vi "3458A Select Aperture.vi"(1 "manual aperture [s]":dbl=1.4e-06 format="%#_6p", 2 "sampling rate [Sa/s]":dbl=10000.0, 3 "digitizer session":T1 {"channels"."Range [Vpk]" min=0.0}) -> (0 "selected aperture [s]":dbl format="%#_6p")   [LabVIEW 2018, in "3458A Virtual Digitizer.lvlib"]
doc: "Auto selection of aperture (if enabled in session!). Otherwise returns input aperture."
uses:
  3458A Virtual Digitizer.lvlib
  3458A Digitizer Session.ctl
  3458A Virtual Channel Config.ctl
  Counter/Counter Session.ctl
  Counter/Counter Type.ctl
  AWG/AWG Session.ctl
  AWG/AWG Type.ctl
  3458A Sync Mode.ctl
  3458A Idn Mode.ctl
  3458A Digitizing Low Levels/Configure/Sampling Mode.ctl
  3458A Digitizing Process Options.ctl
  3458A Data Packet.ctl
  3458A Aux Record Data.ctl
  3458A Digitizing Low Levels/Configure/Level Setup.ctl
  3458A Digitizing Low Levels/Configure/First Sample Trigger.ctl
  3458A Aperture Selection Mode.ctl
  3458A Digitizing Low Levels/3458A Digitizing Low Levels.lvlib
  Counter/Counter.lvlib
  AWG/AWG.lvlib
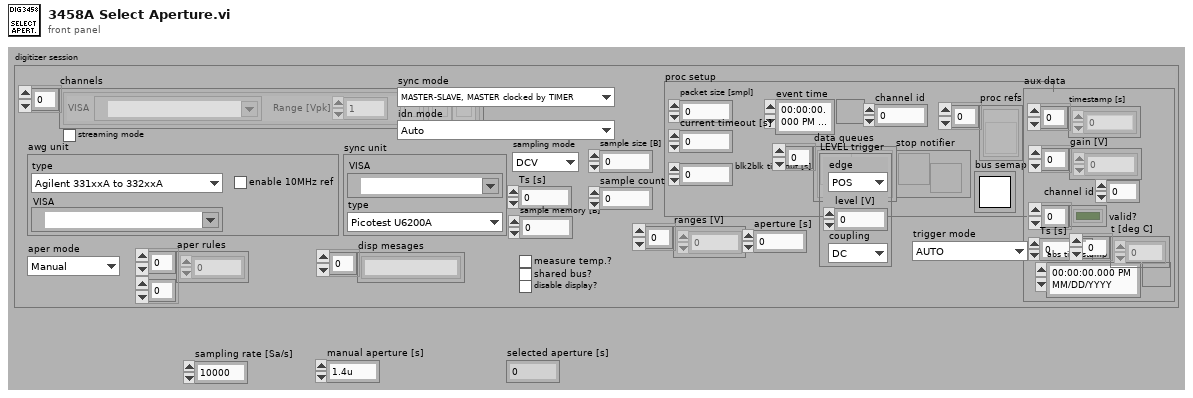
[diagram p1: front panel]
types:
  T1 = typedef "3458A Virtual Digitizer.lvlib/3458A Digitizer Session.ctl" = cluster{"channels":T2[], "sync unit":T3, "awg unit":T5, "sync mode":T7, "streaming mode":bool, "idn mode":T8, "sampling mode":T9, "Ts [s]":dbl, "sample memory [B]":i32, "proc setup":T10, "sample size [B]":i32, "sample count":i32, "aux data":T12, "ranges [V]":dbl[], "aperture [s]":dbl, "LEVEL trigger":T13, "trigger mode":T14, "measure temp.?":bool, "disp mesages":string[], "shared bus?":bool, "disable display?":bool, "aper mode":T15, "aper rules":dbl[][]}
  T2 = typedef "3458A Virtual Digitizer.lvlib/3458A Virtual Channel Config.ctl" = cluster{"VISA":refnum<visa-resource-name>, "Range [Vpk]":dbl, "btn clr":bool, "btn up":bool, "btn down":bool}
  T3 = typedef "Counter.lvlib/Counter Session.ctl" = cluster{"VISA":refnum<visa-resource-name>, "type":T4}
  T4 = typedef "Counter.lvlib/Counter Type.ctl" = enum16{"Picotest U6200A", "dummy"}
  T5 = typedef "AWG.lvlib/AWG Session.ctl" = cluster{"type":T6, "VISA":refnum<visa-resource-name>, "enable 10MHz ref":bool}
  T6 = typedef "AWG.lvlib/AWG Type.ctl" = enum16{"Agilent 331xxA to 332xxA", "Agilent 335xxA to 336xxA", "Tektronix AFG3101C", "dummy"}
  T7 = typedef "3458A Virtual Digitizer.lvlib/3458A Sync Mode.ctl" = enum16{"MASTER-SLAVE, MASTER clocked by TIMER", "MASTER-SLAVE, MASTER clocked by AWG", "ALL clocked by AWG", "MASTER-SLAVE, ALL clocked by TIMER", "ALL clocked by AWG with DFLL"}
  T8 = typedef "3458A Virtual Digitizer.lvlib/3458A Idn Mode.ctl" = enum16{"Auto", "Sequential (chn A, chn B, ...)", "From calibration string"}
  T9 = typedef "3458A Virtual Digitizer.lvlib/3458A Digitizing Low Levels.lvlib/Sampling Mode.ctl" = enum16{"DCV", "DSDC", "DSAC"}
  T10 = typedef "3458A Virtual Digitizer.lvlib/3458A Digitizing Process Options.ctl" = cluster{"channel id":i32, "packet size [smpl]":i32, "current timeout [s]":dbl, "blk2blk timeout [s]":dbl, "event time":timestamp, "stop notifier":refnum<notifier>, "data queues":refnum<queue>[], "proc refs":refnum<vi>[], "bus semaphore":T11}
  T11 = typedef "Semaphore RefNum" = refnum<k1>
  T12 = typedef "3458A Virtual Digitizer.lvlib/3458A Aux Record Data.ctl" = cluster{"channel id":i32, "valid?":bool[], "gain [V]":dbl[], "timestamp [s]":dbl[], "Ts [s]":dbl, "abs timestamp":timestamp, "t [deg C]":dbl[]}
  T13 = typedef "3458A Virtual Digitizer.lvlib/3458A Digitizing Low Levels.lvlib/Level Setup.ctl" = cluster{"edge":enum16{"POS", "NEG"}, "level [V]":dbl, "coupling":enum16{"DC", "AC"}}
  T14 = typedef "3458A Virtual Digitizer.lvlib/3458A Digitizing Low Levels.lvlib/First Sample Trigger.ctl" = enum16{"AUTO", "EXT", "SYN", "SGL", "HOLD", "LEVEL"}
  T15 = typedef "3458A Virtual Digitizer.lvlib/3458A Aperture Selection Mode.ctl" = enum16{"Manual", "Maximum", "Table"}
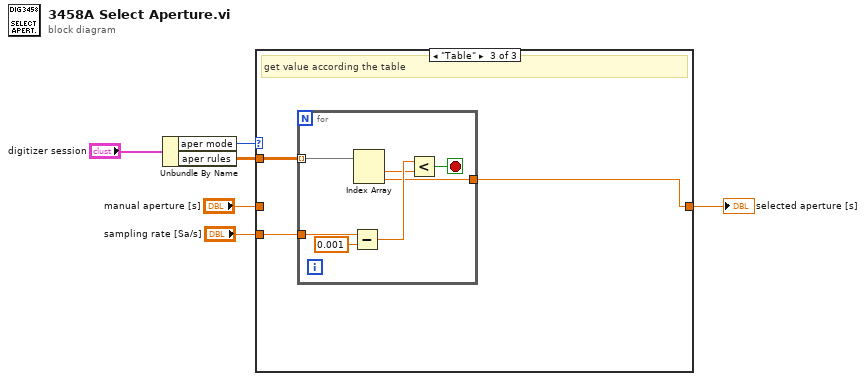
[diagram p0: block diagram]
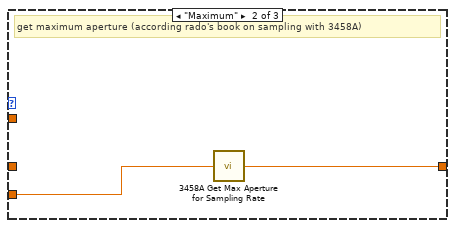
[diagram p3: hidden frame]
diagram:
  n1 = Unbundle By Name("digitizer session") -> ("aper mode"=w5:T15, "aper rules"=w1:dbl[][])
  n2 = case shown="\"Table\"" w5 {
    tunnel: "manual aperture [s]" -> [w7 _ _]
    tunnel: [w7 w9 w10] -> w3
    tunnel: "sampling rate [Sa/s]" -> [_ w8 w11]
    tunnel: w1 -> [_ _ w12]
    frame "Manual", Default {
      # "user entry"
    }
    frame "Maximum" {
      # "get maximum aperture (according rado's book on sampling with 3458A)"
      n3 = call "3458A Get Max Aperture for Sampling Rate.vi"("fs [Hz]"=w8) -> ("ta_max [s]"=w9:dbl)
    }
    frame "Table" {
      # "get value according the table"
      n4 = for {
        tunnel: w12 -> [w19] mode=indexing
        tunnel: w11 -> [w18]
        tunnel: [w14] -> w10
        stop <- w13 stop-if-true
        n5 = Subtract(x=w18, y=0.001) -> (x-y=w16:dbl)
        n6 = Index Array(array=w19) -> (element #1=w15:dbl, element #2=w14:dbl)  [unwired: 2 in]
        n7 = Less?(x=w16, y=w15) -> (x < y?=w13:bool)
      }
    }
  }
  "selected aperture [s]" <- w3
